vi "CONCATENATE STRINGS.vi"() -> ()   [LabVIEW 2019]
panel:
  in  "String 2":string
  in  "String 1":string
  out "Concatenated string":string
  # "CONCATENATE  STRINGS"
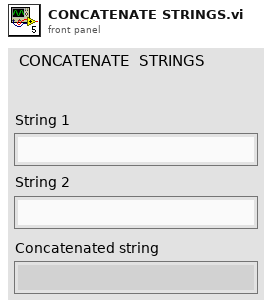
[diagram p1: front panel]
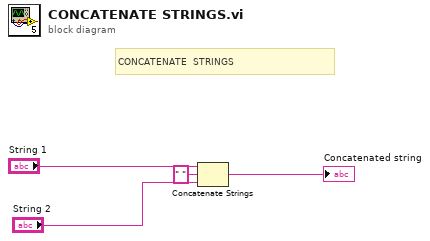
[diagram p0: block diagram]
diagram:
  # "CONCATENATE  STRINGS"
  n1 = Concatenate Strings("String 1", " " ("string"), "String 2") -> (→"Concatenated string":string)
